vi "Freigabe Funktionen schalten.vi"(5 "Samplepoint ALT":u16, 6 "Aktionen":T1, 7 "Samplepoint NEU":u16, 8 "Freigabe?":bool, 10 "Zustand ALT":T2, 11 "Zustand NEU":T2) -> (0 "Freigabe?":bool, 2 "Zustand":T2, 4 "Samplepoint":u16)   [LabVIEW 2020, in "Funktionstasten.lvlib"]
uses:
  Funktionstasten.lvlib
  Zustaende.ctl
  Freigabe Aktionen.ctl
  Allgemein/allgemeine Sub-VIs.lvlib
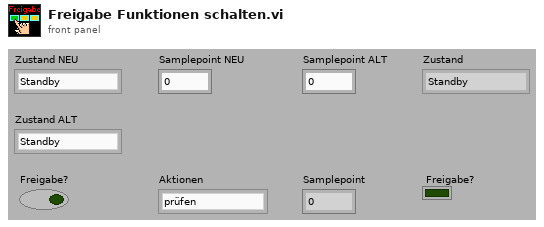
[diagram p1: front panel]
types:
  T1 = typedef "Funktionstasten.lvlib/Freigabe Aktionen.ctl" = enum16{"prüfen", "Freigabe?", "lesen"}
  T2 = typedef "Funktionstasten.lvlib/Zustaende.ctl" = enum16{"Standby", "Pause", "Eco", "Messen", "Kalibrieren", "Spülen Filter", "Spülen Leitung", "Umgebungsluft", "0-Gas", "Cal-Gas", "CG zu PNS", "-------------", "Init 1", "Init 2", "Init 3", "Init 4", "Messen vorbereiten", "Messen durchführen", "Exit"}
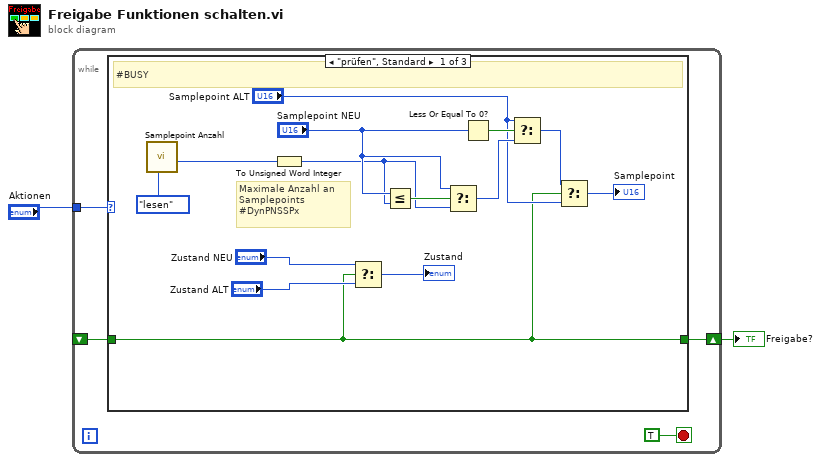
[diagram p0: block diagram]
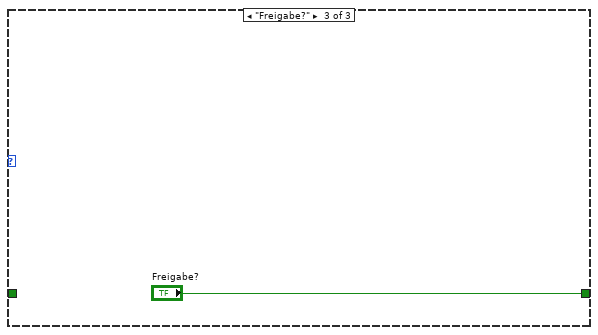
[diagram p3: hidden frame]
diagram:
  n1 = while {
    tunnel: "Aktionen" -> [w6]
    shift-right: [w4] -> w1
    shift-left: _ -> [w3]
    stop <- TRUE stop-if-true
    n2 = case shown="\"prüfen\", Standard" w6 {
      tunnel: [w7 w21 "Freigabe?"] -> w4
      tunnel: w3 -> [w7 w21 _]
      frame "prüfen", Default {
        # "Maximale Anzahl an \nSamplepoints\n#DynPNSSPx"
        # "#BUSY"
        n3 = call "Samplepoint Anzahl.vi"("Aktion"=enum16{"lesen", "Ref schreiben", "SP setzen"}."lesen") -> ("Anzahl SP"=w8:i32)  [unwired: 9 in, 1 out]
        n4 = To Unsigned Word Integer(number=w8) -> (unsigned 16bit integer=w9:u16)
        n5 = Select(t="Zustand NEU", s=w7, f="Zustand ALT") -> (s? t:f=→"Zustand":T2)
        n6 = Less Or Equal?(x="Samplepoint NEU", y=w9) -> (x <= y?=w16:bool)
        n7 = Select(t="Samplepoint NEU", s=w16, f=w9) -> (s? t:f=w14:u16)
        n8 = Less Or Equal To 0?(x="Samplepoint NEU") -> (x <= 0?=w15:bool)
        n9 = Select(t="Samplepoint ALT", s=w15, f=w14) -> (s? t:f=w12:u16)
        n10 = Select(t=w12, s=w7, f="Samplepoint ALT") -> (s? t:f=→"Samplepoint":u16)
      }
      frame "lesen" {
        # "#BUSY"
      }
      frame "Freigabe?" {
      }
    }
  }
  "Freigabe?" <- w1
